vi "channel_consumer.vi"(4 "timeout":i32=100, 5 "error in":errorcluster, 7 "TDMS channel":T1, 8 "TDMS in":refnum<k34>) -> (0 "error out":errorcluster, 2 "count":i32, 3 "TDMS out":refnum<k34>)   [LabVIEW 2020]
uses:
  <extravilib>/ChannelInstances/Messenger-c(str,a[.](str),var)/))Channel.ctl
  <extravilib>/ChannelInstances/Messenger-c(str,a[.](str),var)/Read With Abort.vi
  <extravilib>/ChannelInstances/Messenger-c(str,a[.](str),var)/Endpoint.vi
  <extravilib>/ChannelInstances/Messenger-c(str,a[.](str),var).lvlib
  <vilib>/Utility/Data Type/NI_Data Type.lvlib
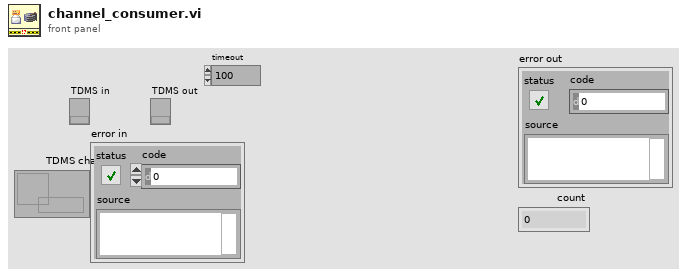
[diagram p1: front panel]
types:
  T1 = typedef "Messenger-c(str,a[.](str),var).lvlib/))Channel.ctl" = refnum<queue>
  T2 = typedef "NI_Data Type.lvlib/Data Type.ctl" = enum8{"Invalid Type", "Void", "I8", "I16", "I32", "I64", "U8", "U16", "U32", "U64", "Single Float", "Double Float", "Extended Float", "Single Complex", "Double Complex", "Extended Complex", "Enum U8", "Enum U16", "Enum U32", "Enum U64", "Single Float With Unit", "Double Float With Unit", "Extended Float With Unit", "Single Complex with Unit", "Double Complex with Unit", "Extended Complex with Unit", "Boolean", "String", "Path", "Picture", "Tag", "Array", "Cluster", "Variant", "LV Variant", "Waveform", "Timestamp", "Digital Waveform", "Digital Data", "ExpressData", "Refnum", "External Data", "VI", "Poly VI", "LabVIEW Class Instance", "Fixed Point", "Set Collection", "Map Collection"}
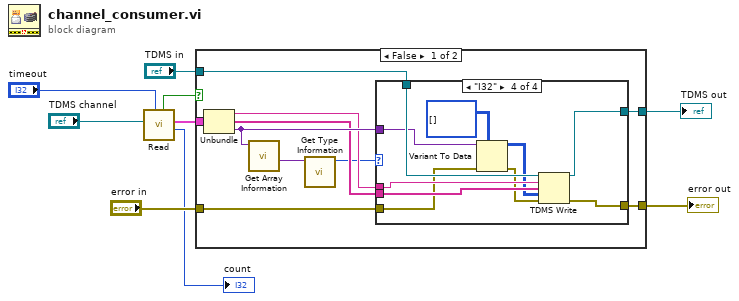
[diagram p0: block diagram]
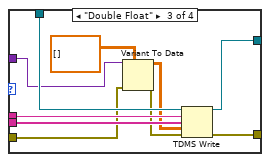
[diagram p4: hidden frame]
diagram:
  n1 = call <extravilib>:"Read.vi"("timeout in ms (-1)"="timeout", "channel"="TDMS channel") -> ("remaining"=→"count":i32, "element"=w9:cluster{string, string[], "Variant":variant}, "timed out?"=w2:bool)  [unwired: 7 in]
  n2 = case shown="False" w2 {
    tunnel: w9 -> [w14 _]
    tunnel: "TDMS in" -> [w13 w45]
    tunnel: [w12 w45] -> w6
    tunnel: "error in" -> [w11 w44]
    tunnel: [w10 w44] -> w4
    frame False {
      n3 = Unbundle(w14) -> (w17:string, w18:string[], "Variant"=w19:variant)
      n4 = call <vilib>:"Get Array Information.vi"("variant"=w19) -> ("array element data type"=w15:variant)  [unwired: 7 in, 3 out]
      n5 = call <vilib>:"Get Type Information.vi"("variant"=w15) -> ("type"=w16:T2)  [unwired: 6 in, 4 out]
      n6 = case shown="\"I32\"" w16 {
        tunnel: w13 -> [w21 w23 w33 w43]
        tunnel: w17 -> [_ _ w32 w42]
        tunnel: w18 -> [_ _ w31 w41]
        tunnel: [w21 w23 w30 w40] -> w12
        tunnel: w19 -> [_ _ w28 w39]
        tunnel: w11 -> [w20 w22 w24 w35]
        tunnel: [w20 w22 w26 w34] -> w10
        frame "Invalid Type", Default {
        }
        frame "Void" {
        }
        frame "Double Float" {
          n7 = Variant To Data(error in=w24, type=dbl[][] [], Variant=w28) -> (data=w27:dbl[][], error out=w25:errorcluster)
          n8 = TDMS Write(0:w33, 5:w32, 7:w31, 9:w27, 11:w25) -> (4:w30:refnum<k34>, 15:w26:errorcluster)  [unwired: 1 in, 2 out]
        }
        frame "I32" {
          n9 = Variant To Data(error in=w35, type=i32[][] [], Variant=w39) -> (data=w37:i32[][], error out=w36:errorcluster)
          n10 = TDMS Write(0:w43, 5:w42, 7:w41, 9:w37, 11:w36) -> (4:w40:refnum<k34>, 15:w34:errorcluster)  [unwired: 1 in, 2 out]
        }
      }
    }
    frame True {
    }
  }
  "TDMS out" <- w6
  "error out" <- w4
